vi "DWF FGEN Init DtoA.vi"() -> (0 "Error Out":errorcluster, 3 "Instrument Handle Out":u32)   [LabVIEW 2025]
uses:
  <vilib>/DigilentWF/FGEN/WF-FGEN.lvlib
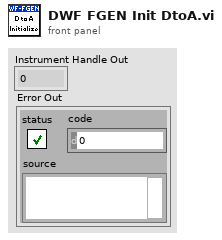
[diagram p1: front panel]
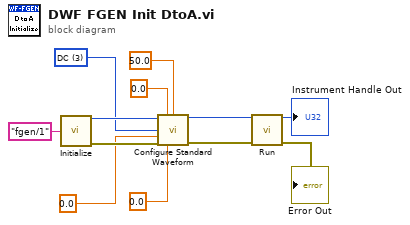
[diagram p0: block diagram]
diagram:
  w5 = 3 items=["Sine", "Square", "Triangle/Ramp", "DC"] ("Waveform Function")
  n1 = call <vilib>:"Initialize.vi"("Channel"="fgen/1") -> ("Instrument Handle Out"=w10:i32, "Error Out"=w11:errorcluster)  [unwired: 13 in]
  n2 = call <vilib>:"Configure Standard Waveform.vi"("Instrument Handle In"=w10, "Frequency"=0.0, "Duty Cycle"=50.0, "Waveform Function"=w5, "Amplitude"=0.0, "Error In"=w11, "DC Offset"=0.0) -> ("Instrument Handle Out"=w8:i32, "Error Out"=w9:errorcluster)  [unwired: 7 in]
  n3 = call <vilib>:"Run.vi"("Instrument Handle In"=w8, "Error In"=w9) -> ("Instrument Handle Out"=→"Instrument Handle Out":i32, "Error Out"=→"Error Out":errorcluster)  [unwired: 12 in]
